vi "constants.vi"() -> ()   [LabVIEW 2020]
doc: "These global variables store constant values configured in Begin."
panel:
  out "Legal_Actuator_Names":string[](array[string])
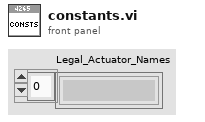
[diagram p1: front panel]
diagram:
